vi "생산 소비자 데이터.vi"() -> ()   [LabVIEW 2019]
panel:
  in  "데이터 전달":bool
  in  "정지":bool
  out "수신 데이터":cluster{"이름":string, "토익 점수":dbl}
  in  "송신 데이터":cluster{"이름":string, "토익 점수":dbl}
  out "소비 루프 반복 횟수":i32
  out "생산 루프 반복 횟수":i32
  # "전달"
  # "전달하지 않음"
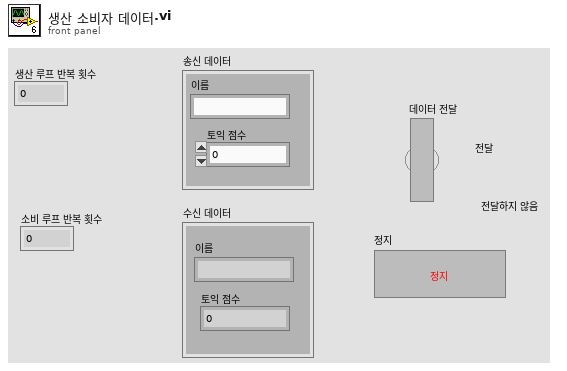
[diagram p1: front panel]
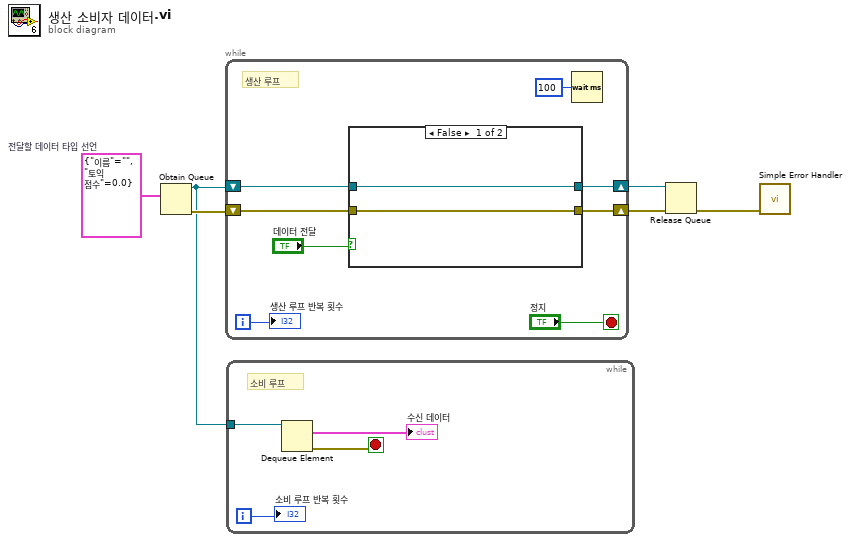
[diagram p0: block diagram]
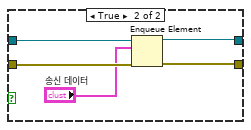
[diagram p2: hidden frame]
diagram:
  w2 = cluster{"이름":string, "토익 점수":dbl} {"이름"="", "토익 점수"=0.0}  # 전달할 데이터 타입 선언
  n1 = Obtain Queue(element data type=w2) -> (queue out=w1:refnum<queue>, error out=w3:errorcluster)  [unwired: 4 in, 1 out]
  n2 = while {
    shift-right: [w10] -> w6
    shift-left: w1 -> [w12]
    shift-right: [w9] -> w5
    shift-left: w3 -> [w11]
    i -> [w14]
    stop <- "정지" stop-if-true
    # "생산 루프"
    n3 = case shown="False" "데이터 전달" {
      tunnel: w12 -> [w16 w19]
      tunnel: w11 -> [w15 w18]
      tunnel: [w16 w21] -> w10
      tunnel: [w15 w20] -> w9
      frame False {
      }
      frame True {
        n4 = Enqueue Element(queue=w19, element="송신 데이터", error in (no error)=w18) -> (queue out=w21:refnum<queue>, error out=w20:errorcluster)  [unwired: 1 in, 1 out]
      }
    }
    n5 = Wait (ms)(milliseconds to wait=u32 100) -> ()  [unwired: 1 out]
    "생산 루프 반복 횟수" <- w14
  }
  n6 = while {
    tunnel: w1 -> [w22]
    i -> [w25]
    stop <- w24 stop-if-true
    # "소비 루프"
    n7 = Dequeue Element(queue=w22) -> (element=→"수신 데이터":cluster{"이름":string, "토익 점수":dbl}, error out=w24:errorcluster)  [unwired: 2 in, 2 out]
    "소비 루프 반복 횟수" <- w25
  }
  n8 = Release Queue(queue=w6, error in (no error)=w5) -> (error out=w4:errorcluster)  [unwired: 1 in, 2 out]
  n9 = call <vilib>:"Simple Error Handler.vi"("error in (no error)"=w4) -> ()  [unwired: 4 in, 5 out]
